vi "Filter String_Handler.vi"(5 "Disable":bool, 6 "Text Colors":T1={"Enabled Color"=0, "Disabled Color"=10395294}, 7 "Make key focus?":bool, 10 "Default Value":string="Filter...", 11 "String Ref":refnum<vi>) -> ()   [LabVIEW 2023]
doc: "Called asynchronously, this VI sets the default string (default=\"Filter...\") and the secondary color to the control's text color (default = gray), then monitors the control for a change in focus. When control gains focus, it removes the default string and sets the text to the main text color. When it loses focus, and if string is empty, it sets the value to the default and sets secondary text color.\n\nMake key focus will place the cursor before the default text and handle removing default text if user types any ascii character"
panel:
  in  "Debug String":string
  # "Debug control:"
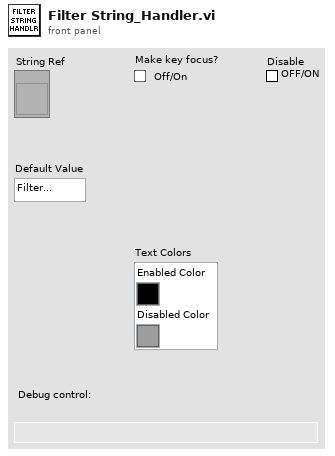
[diagram p1: front panel]
types:
  T1 = cluster{"Enabled Color":u32, "Disabled Color":u32}
  T2 = enum8{"Enabled", "Disabled", "Disabled and Grayed Out"}
  T3 = cluster{"Selection Start":u32, "Selection End":u32}
  T4 = typedef "eventvkey.ctl" = enum16{"ASCII", "Enter", "Return", "Shift", "Ctrl", "Alt", "Cmd", "Opt", "Caps", "NumLock", "Clear", "Break", "Up", "Down", "Left", "Right", "Insert", "Delete", "Home", "End", "PageUp", "PageDown", "Escape", "Help", "Pause", "ScrollLock", "F1", "F2", "F3", "F4", "F5", "F6", "F7", "F8", "F9", "F10", "F11", "F12", "F13", "F14", "F15", "F16", "F17", "F18", "F19", "F20", "F21", "F22", "F23", "F24", "Play", "VolumeUp", "VolumeDown", "Mute", "Two Byte Char"}
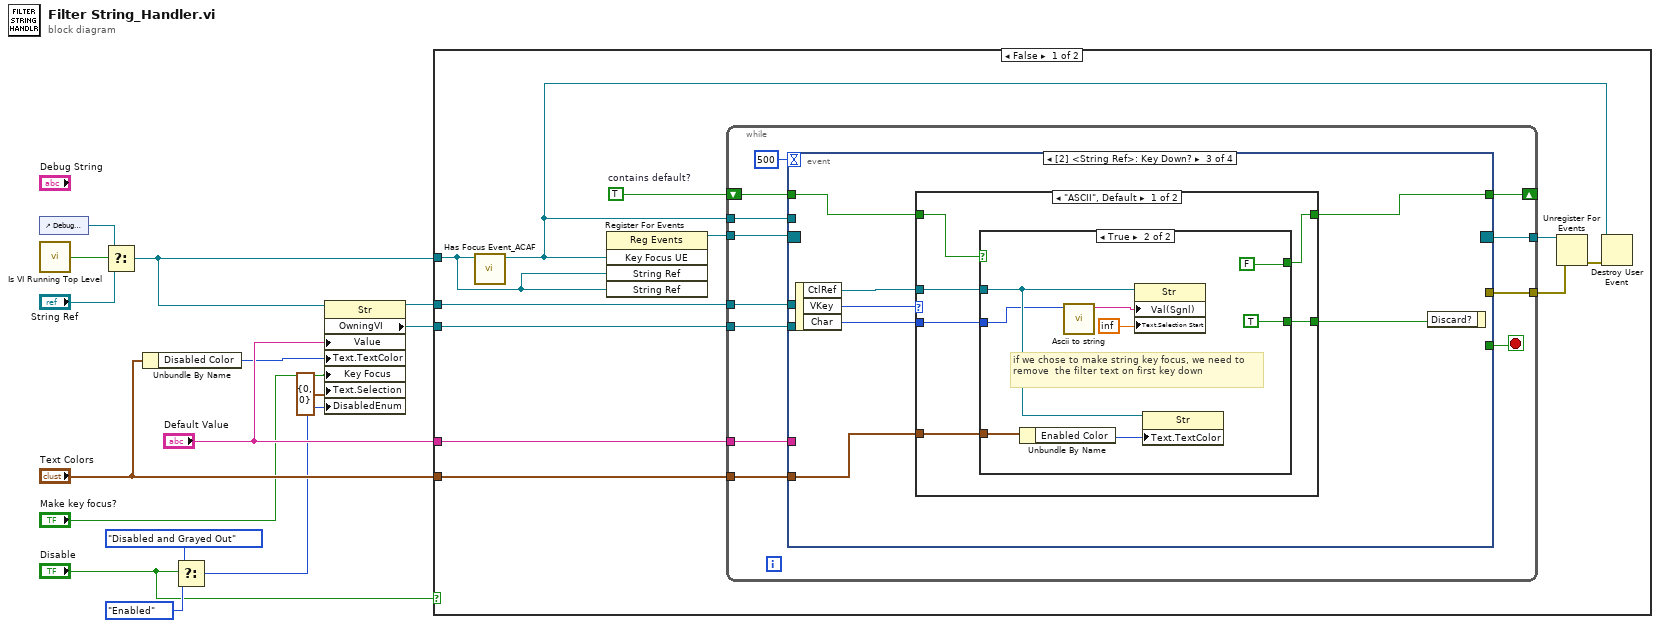
[diagram p0: block diagram]
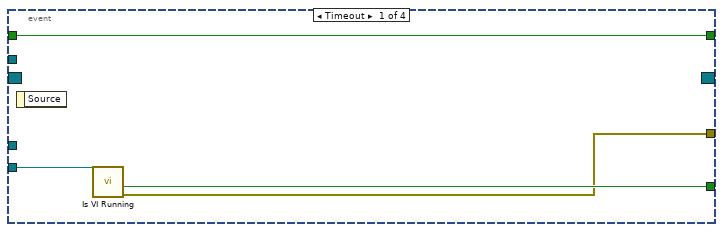
[diagram p2: hidden frame]
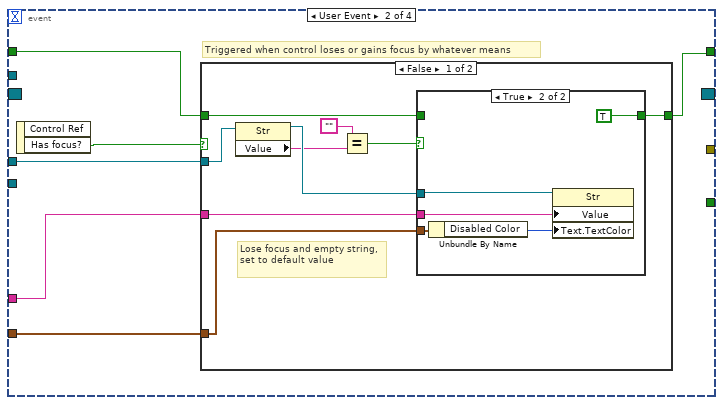
[diagram p3: hidden frame]
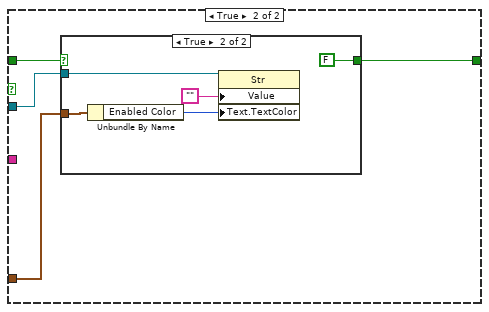
[diagram p5: hidden frame]
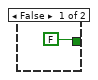
[diagram p7: hidden frame]
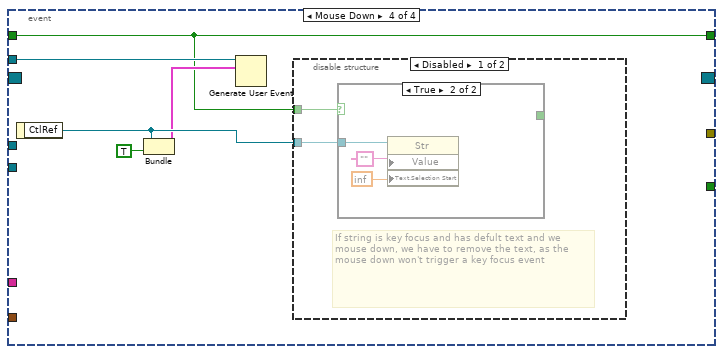
[diagram p9: hidden frame]
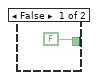
[diagram p10: hidden frame]
diagram:
  n1 = control-ref of="Debug String"() -> (w14:refnum<vi>)
  n2 = call "Is VI Running Top Level.vi"() -> ("Top Level?"=w15:bool)  [unwired: 5 in]
  n3 = Select(t=w14, s=w15, f="String Ref") -> (s? t:f=w2:refnum<vi>)
  n4 = Unbundle By Name("Text Colors") -> ("Disabled Color"=w9:u32)
  n5 = Select(t=T2."Disabled and Grayed Out" ("Disabled"), s="Disable", f=T2."Enabled" ("Disabled")) -> (s? t:f=w3:T2)
  n6 = property class="Str"(reference=w2, "Value"="Default Value", "Text.TextColor"=w9, "Key Focus"="Make key focus?", "Text.Selection"=T3 {"Selection Start"=0, "Selection End"=0}, "DisabledEnum"=w3) -> (reference out=w8:refnum<vi>, "OwningVI"=w11:refnum<vi>)  [unwired: 1 in, 1 out]
  n7 = case shown="False" "Disable" {
    tunnel: "Text Colors" -> [w25 _]
    tunnel: w11 -> [w24 _]
    tunnel: "Default Value" -> [w22 _]
    tunnel: w8 -> [w21 _]
    tunnel: w2 -> [w17 _]
    frame False {
      w23 = TRUE  # contains default?
      n8 = call "Has Focus Event_ACAF.vi"("Control Ref"=w17) -> ("Key Focus UE"=w16:refnum<user-event>)  [unwired: 9 in, 1 out]
      n9 = register-events(w16, w17, w17) -> (reference out=w26:refnum<event-registration>)  [unwired: 2 in, 1 out]
      n10 = while {
        tunnel: w26 -> [w36]
        tunnel: w22 -> [w35]
        tunnel: w25 -> [w34]
        tunnel: w24 -> [w33]
        shift-right: [w31] -> _
        shift-left: w23 -> [w32]
        tunnel: [w30] -> w19
        tunnel: w21 -> [w29]
        tunnel: [w28] -> w20
        tunnel: w16 -> [w27]
        stop <- w38 stop-if-true
        n11 = event shown="[2] <String Ref>: Key Down?" {
          selector: w36 -> [_ _ _ _]
          dyn-events: [_ _ _ _] -> w28
          timeout: 500 -> [_ _ _ _]
          tunnel: [w41 _ _ _] -> w38
          tunnel: w35 -> [_ w47 _ _]
          tunnel: w34 -> [_ w46 w75 _]
          tunnel: w33 -> [w42 _ _ _]
          tunnel: [w40 w44 w80 w97] -> w31
          tunnel: w32 -> [w40 w45 w79 w97]
          tunnel: [w39 _ _ _] -> w30
          tunnel: w29 -> [_ w43 _ _]
          tunnel: w27 -> [_ _ _ w101]
          event Timeout {
            n12 = event-data() -> ()  [unwired: 1 in, 1 out]
            n13 = call "Is VI Running.vi"("VI in"=w42) -> ("error out"=w39:errorcluster, "VI Not Running"=w41:bool)  [unwired: 7 in, 2 out]
          }
          event User Event {
            # "Triggered when control loses or gains focus by whatever means"
            n14 = event-data() -> ("Has focus?"=w48:bool)  [unwired: 1 in, 1 out]
            n15 = case shown="False" w48 {
              tunnel: w47 -> [w54 _]
              tunnel: w46 -> [w53 w67]
              tunnel: w45 -> [w49 w66]
              tunnel: [w52 w65] -> w44
              tunnel: w43 -> [w50 w64]
              frame False {
                # "Lose focus and empty string, set to default value"
                n16 = property class="Str"(reference=w50) -> (reference out=w56:refnum<vi>, "Value"=w51:string)  [unwired: 1 in, 1 out]
                n17 = Equal?(x="", y=w51) -> (x = y?=w55:bool)
                n18 = case shown="True" w55 {
                  tunnel: w56 -> [_ w59]
                  tunnel: w54 -> [_ w63]
                  tunnel: w53 -> [_ w62]
                  tunnel: [w58 TRUE] -> w52
                  tunnel: w49 -> [w58 _]
                  frame False {
                  }
                  frame True {
                    n19 = Unbundle By Name(w62) -> ("Disabled Color"=w61:u32)
                    n20 = property class="Str"(reference=w59, "Value"=w63, "Text.TextColor"=w61) -> ()  [unwired: 1 in, 2 out]
                  }
                }
              }
              frame True {
                n21 = case shown="True" w66 {
                  selector: w66 -> [w68 _]
                  tunnel: w64 -> [_ w72]
                  tunnel: w67 -> [_ w71]
                  tunnel: [w68 FALSE] -> w65
                  frame False {
                  }
                  frame True {
                    n22 = Unbundle By Name(w71) -> ("Enabled Color"=w70:u32)
                    n23 = property class="Str"(reference=w72, "Value"="", "Text.TextColor"=w70) -> ()  [unwired: 1 in, 2 out]
                  }
                }
              }
            }
          }
          event Key Down? {
            n24 = event-data() -> ("CtlRef"=w77:refnum<vi>, "VKey"=w78:T4, "Char"=w74:i16)  [unwired: 1 in]
            n25 = case shown="\"ASCII\", Default" w78 {
              tunnel: [w85 w96] -> w80
              tunnel: w79 -> [w86 w96]
              tunnel: w77 -> [w84 _]
              tunnel: [w83 _] -> w76
              tunnel: w75 -> [w82 _]
              tunnel: w74 -> [w81 _]
              frame "ASCII", Default {
                n26 = case shown="True" w86 {
                  tunnel: [FALSE FALSE] -> w85
                  tunnel: w84 -> [_ w91]
                  tunnel: [_ TRUE] -> w83
                  tunnel: w82 -> [_ w90]
                  tunnel: w81 -> [_ w88]
                  frame False {
                  }
                  frame True {
                    # "if we chose to make string key focus, we need to remove  the filter text on first key down"
                    n27 = Unbundle By Name(w90) -> ("Enabled Color"=w92:u32)
                    n28 = call "Ascii to string.vi"("ASCII Code"=w88) -> ("String"=w89:string)  [unwired: 10 in]
                    n29 = property class="Str"(reference=w91, "Val(Sgnl)"=w89, "Text.Selection Start"=inf) -> ()  [unwired: 1 in, 2 out]
                    n30 = property class="Str"(reference=w91, "Text.TextColor"=w92) -> ()  [unwired: 1 in, 2 out]
                  }
                }
              }
              frame "Enter" {
              }
            }
            n31 = event-data("Discard?"=w76) -> ()  [unwired: 1 in, 1 out]
          }
          event Mouse Down {
            n32 = event-data() -> ("CtlRef"=w100:refnum<vi>)  [unwired: 1 in]
            n33 = Bundle("CtlRef"=w100, TRUE) -> (w99:cluster{"CtlRef":refnum<vi>, bool})  [unwired: 1 in]
            n34 = Generate User Event(user event=w101, event data cluster=w99) -> ()  [unwired: 2 in, 2 out]
            n35 = disable-structure shown="Disabled" {
              disable-tunnel: w97 -> [w103 _]
              disable-tunnel: w100 -> [w102 _]
              frame Disabled {
                # "If string is key focus and has defult text and we mouse down, we have to remove the text, as the mouse down won't trigger a key focus event"
                n36 = case shown="True" w103 {
                  tunnel: [FALSE _] -> _
                  tunnel: w102 -> [_ w107]
                  frame False {
                  }
                  frame True {
                    n37 = property class="Str"(reference=w107, "Value"="", "Text.Selection Start"=inf) -> ()  [unwired: 1 in, 2 out]
                  }
                }
              }
              frame Enabled {
              }
            }
          }
        }
      }
      n38 = Unregister For Events(event registration refnum=w20, error in=w19) -> (error out=w18:errorcluster)
      n39 = Destroy User Event(user event=w16, error in=w18) -> ()  [unwired: 1 out]
    }
    frame True {
    }
  }
